vi "pdpterminals.vi"() -> ()   [LabVIEW 2019]
panel:
  out "Wheel_3_Azimuth":i32
  out "Wheel_2_Azimuth":i32
  out "Wheel_1_Azimuth":i32
  out "Wheel_0_Azimuth":i32
  out "Wheel_3_Speed":i32
  out "Wheel_2_Speed":i32
  out "Wheel_1_Speed":i32
  out "Wheel_0_Speed":i32
  # "--drive subsystem--"
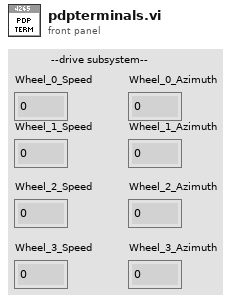
[diagram p1: front panel]
diagram:
